vi "Cleanup.vi"(8 "error in (no error)":errorcluster, 11 "Node in":refnum<class "bt_Node.lvclass">) -> (0 "error out":errorcluster, 3 "Node out":refnum<class "bt_Node.lvclass">)   [LabVIEW 2021, in "BT.lvlib" / "bt_Node.lvclass"]
uses:
  bt_Node.lvclass
  bt_Node.lvclass/bt_Node.ctl
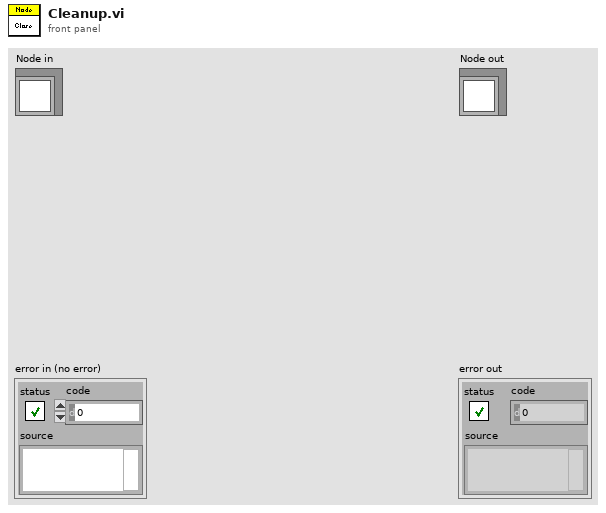
[diagram p1: front panel]
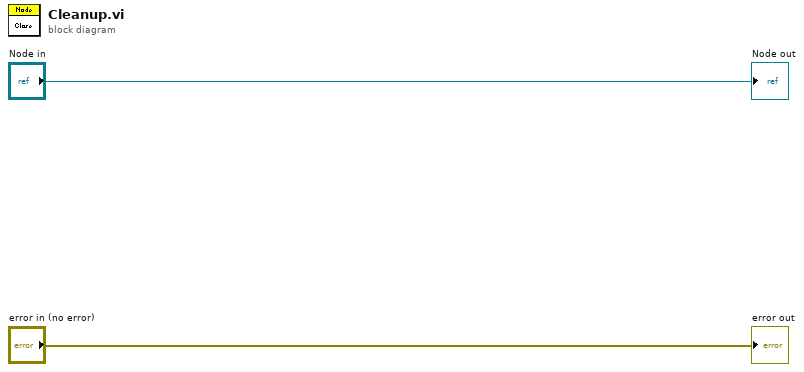
[diagram p0: block diagram]
diagram:
  "error out" <- "error in (no error)"
  "Node out" <- "Node in"
